vi "simulacion - copia.vi"() -> ()   [LabVIEW 2018]
uses:
  <vilib>/platform/TimedLoop/XDataNode/XDataNode.xnode
  <vilib>/Platform/TimedLoop/XDataNode/nitl_modes.ctl
  <vilib>/Platform/TimedLoop/XDataNode/XDNodeRunTimeDep.lvlib
  <vilib>/Platform/TimedLoop/XDataNode/wakeup.ctl
  <vilib>/Platform/TimedLoop/XDataNode/timing_clust.ctl
  <vilib>/Analysis/Matrix/NI_Matrix.lvlib
  <vilib>/Analysis/Matrix/Numeric/Conversions/Array To Matrix - RA2.vi
  <vilib>/Analysis/Matrix/Numeric/Add/Add - RM,RM.vi
  <vilib>/Analysis/Matrix/Datatypes/RealMatrix.ctl
  <vilib>/Analysis/Matrix/Numeric/Conversions/Array To Matrix - RA.vi
  <vilib>/Analysis/Matrix/Numeric/Multiply/Multiply - RM,RM.vi
panel:
  out "element":dbl
  out "A + B":T1
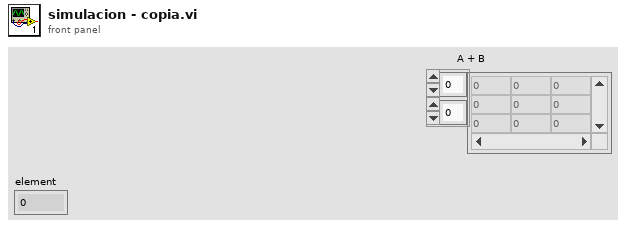
[diagram p1: front panel]
types:
  T1 = typedef "NI_Matrix.lvlib/RealMatrix.ctl" = dbl[][]
  T2 = typedef "XDNodeRunTimeDep.lvlib/timing_clust.ctl" = cluster{"Expected End [f-1]":u64, "Actual End [f-1]":u64, "Finished Late? [f-1]":bool, "Expected End [i-1]":u64, "Actual End [i-1]":u64, "Finished Late? [i-1]":bool, "Expected Start [i]":u64, "Actual Start [i]":u64, "Expected Start [f]":u64, "Actual Start [f]":u64, "Source Name":string, "Structure Name":string, "Period":i64, "Deadline":i64, "Offset":i64, "Start":i64, "Priority":i32, "Timeout":i32, "Mode":T3, "Wakeup Reason":T4, "Error":errorcluster, "Source Type":string, "Secondary Source Type":string, "Global End Time":u64, "Global Start Time":u64, "Frame Duration":u64, "Iteration Duration":u64, "Assigned CPU":i32, "I/O Scan Engine Mode":u32}
  T3 = typedef "XDNodeRunTimeDep.lvlib/nitl_modes.ctl" = enum32{"No Change", "Process missed periods, maintain original phase", "Discard missed periods, maintain original phase", "Process missed periods, ignore original phase", "Discard missed periods, ignore original phase"}
  T4 = typedef "XDNodeRunTimeDep.lvlib/wakeup.ctl" = enum32{"Normal", "Aborted", "Asynchronous wakeup", "Timing source error", "Timed loop error", "Timeout"}
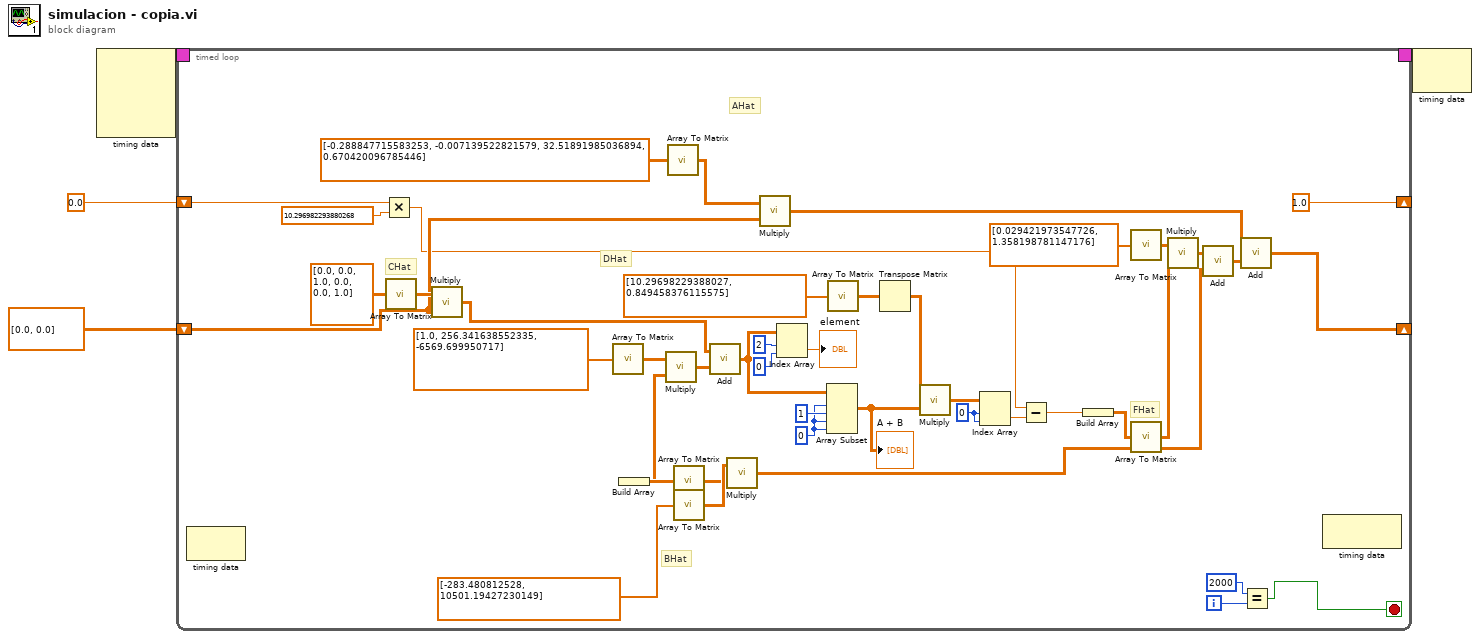
[diagram p0: block diagram]
diagram:
  n1 = node-c288() -> (w4:T2)  [unwired: 4 in]
  n2 = timed-loop {
    timing: w4 -> [_]
    timing-out: [_] -> w3
    shift-right: [1.0] -> _
    shift-left: 0.0 -> [w12]
    shift-right: [w41] -> _
    shift-left: T1 [[0.0], [0.0]] ("A + B") -> [w22]
    i -> [w16]
    stop <- w14 stop-if-true
    w42 = 0 ("index (row)")
    w44 = 0 ("row 1")
    # "DHat"
    # "CHat"
    # "FHat"
    # "AHat"
    # "BHat"
    n3 = node-c288() -> ()  [unwired: 1 in, 1 out]
    n4 = Multiply ("Multiply.vi")(x=w12, y=10.296982293880268) -> (x*y=w10:dbl)
    n5 = call-poly <vilib>:"Array To Matrix.vi"("Real 2D Array"=dbl[][] [[0.0, 0.0], [1.0, 0.0], [0.0, 1.0]]) -> ("Real Matrix"=w23:T1)
    n6 = call-poly <vilib>:"Multiply.vi"("Real Matrix B"=w22, "Real Matrix A"=w23) -> ("A * B"=w21:T1)
    n7 = call-poly <vilib>:"Array To Matrix.vi"("Real 1D Array"=dbl[] [1.0, 256.341638552335, -6569.699950717] ("element")) -> ("Real Matrix (Column Vector)"=w33:T1)
    n8 = Build Array() -> (w46:T1, w5:dbl[])
    n9 = call-poly <vilib>:"Array To Matrix.vi"("Real 2D Array"=dbl[][] [[-0.288847715583253, -0.007139522821579], [32.51891985036894, 0.670420096785446]] ("element")) -> ("Real Matrix"=w32:T1)
    n10 = call-poly <vilib>:"Array To Matrix.vi"("Real 2D Array"=w46) -> ("Real Matrix"=w26:T1)
    n11 = call-poly <vilib>:"Multiply.vi"("Real Matrix B"=w26, "Real Matrix A"=w33) -> ("A * B"=w24:T1)
    n12 = call-poly <vilib>:"Array To Matrix.vi"("Real 1D Array"=dbl[] [-283.480812528, 10501.19427230149] ("element")) -> ("Real Matrix (Column Vector)"=w27:T1)
    n13 = call-poly <vilib>:"Add.vi"("Real Matrix B"=w24, "Real Matrix A"=w21) -> ("A + B"=w9:T1)
    n14 = call-poly <vilib>:"Multiply.vi"("Real Matrix B"=w26, "Real Matrix A"=w27) -> ("A * B"=w25:T1)
    n15 = call-poly <vilib>:"Multiply.vi"("Real Matrix B"=w22, "Real Matrix A"=w32) -> ("A * B"=w31:T1)
    n16 = Index Array(array=w9, index (row)=2, index (col)=0) -> (element=→"element":dbl)
    n17 = Array Subset(array=w9, index (row)=w44, length (row)=1 ("row N"), index (col)=w44, length (col)=w44) -> (w19:T1)
    "A + B" <- w19
    n18 = call-poly <vilib>:"Array To Matrix.vi"("Real 1D Array"=dbl[] [10.29698229388027, 0.849458376115575] ("element")) -> ("Real Matrix (Column Vector)"=w43:T1)
    n19 = Transpose Matrix(1:w43) -> (0:w20:T1)
    n20 = call-poly <vilib>:"Multiply.vi"("Real Matrix B"=w19, "Real Matrix A"=w20) -> ("A * B"=w18:T1)
    n21 = Index Array(array=w18, index (row)=w42, index (col)=w42) -> (element=w13:dbl)
    n22 = Subtract(x=w10, y=w13) -> (x-y=w39:dbl)
    n23 = Build Array(w39) -> (w47:T1)
    n24 = call-poly <vilib>:"Array To Matrix.vi"("Real 1D Array"=dbl[] [0.029421973547726, 1.358198781147176] ("element")) -> ("Real Matrix (Column Vector)"=w30:T1)
    n25 = call-poly <vilib>:"Array To Matrix.vi"("Real 2D Array"=w47) -> ("Real Matrix"=w29:T1)
    n26 = call-poly <vilib>:"Multiply.vi"("Real Matrix B"=w29, "Real Matrix A"=w30) -> ("A * B"=w28:T1)
    n27 = call-poly <vilib>:"Add.vi"("Real Matrix B"=w25, "Real Matrix A"=w28) -> ("A + B"=w40:T1)
    n28 = call-poly <vilib>:"Add.vi"("Real Matrix B"=w40, "Real Matrix A"=w31) -> ("A + B"=w41:T1)
    n29 = Equal?(x=2000, y=w16) -> (x = y?=w14:bool)
    n30 = node-c288() -> ()  [unwired: 1 in, 1 out]
  }
  n31 = node-c288(w3) -> ()  [unwired: 1 out]
